vi "Clean_Up_Template.vi"(1 "Template Info In":string[](array[string])) -> (0 "Template Info Out":string[](array[string]))   [LabVIEW 2018]
uses:
  Controls/Global_mode.ctl
panel:
  in  "Mode":T1
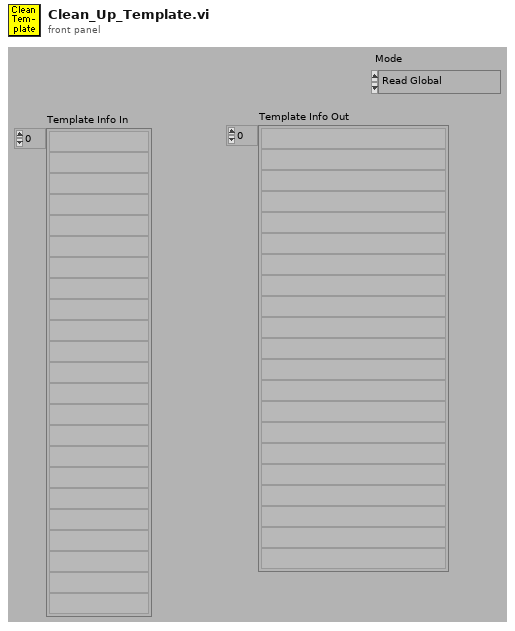
[diagram p1: front panel]
types:
  T1 = typedef "Global_mode.ctl" = enum16{"Read Global", "Load Global From File", "Write Global to File"}
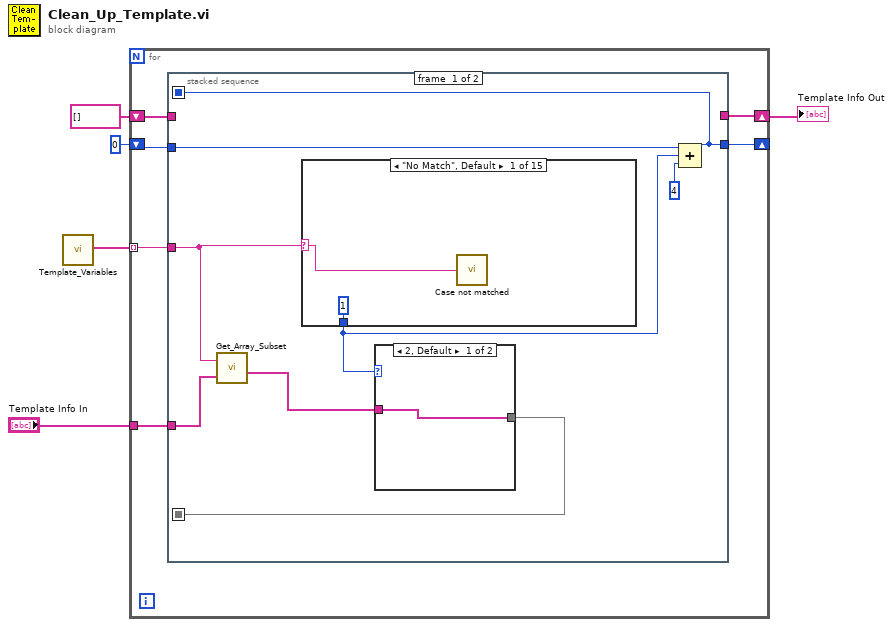
[diagram p0: block diagram]
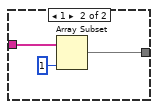
[diagram p2: hidden frame]
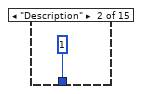
[diagram p3: hidden frame]
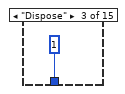
[diagram p4: hidden frame]
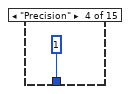
[diagram p5: hidden frame]
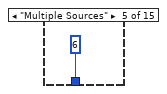
[diagram p6: hidden frame]
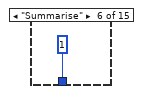
[diagram p7: hidden frame]
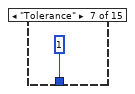
[diagram p8: hidden frame]
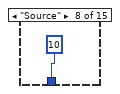
[diagram p9: hidden frame]
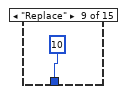
[diagram p10: hidden frame]
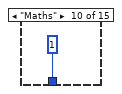
[diagram p11: hidden frame]
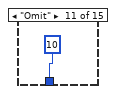
[diagram p12: hidden frame]
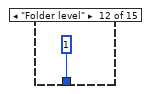
[diagram p13: hidden frame]
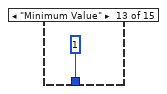
[diagram p14: hidden frame]
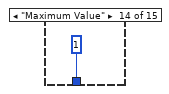
[diagram p15: hidden frame]
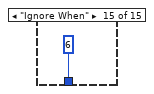
[diagram p16: hidden frame]
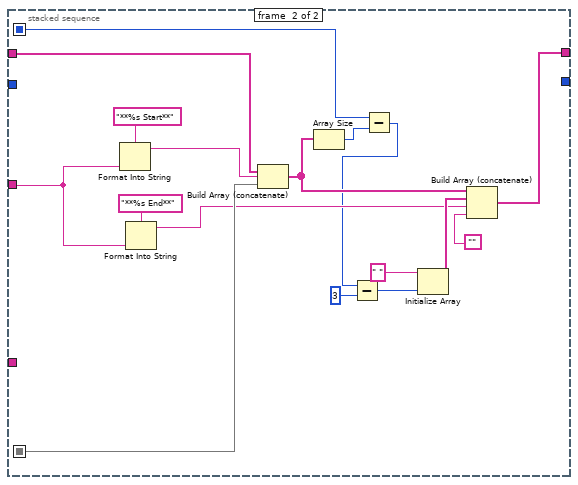
[diagram p17: hidden frame]
diagram:
  n1 = call "Template_Variables.vi"() -> ("Variable Names"=w1:string[])
  n2 = for {
    shift-right: [w6] -> w2
    shift-left: string[] [] -> [w7]
    tunnel: w1 -> [w11] mode=indexing
    tunnel: "Template Info In" -> [w10]
    shift-right: [w8] -> _
    shift-left: 0 -> [w9]
    n3 = stacked-sequence {
      seq-local: [w16 _] -> [_ w51]
      seq-local: [w12 _] -> [_ w49]
      tunnel: w11 -> [w18 w54]
      tunnel: w10 -> [w19 _]
      tunnel: w9 -> [w15 _]
      tunnel: [w12 _] -> w8
      tunnel: w7 -> [_ w53]
      tunnel: [_ w46] -> w6
      frame #0 {
        n4 = call "Get_Array_Subset.vi"("String Array In"=w19, "Subset Name"=w18) -> ("Array Subset Out"=w17:string[])  [unwired: 4 out]
        n5 = case shown="\"No Match\", Default" w18 {
          selector: w18 -> [w24 _ _ _ _ _ _ _ _ _ _ _ _ _ _]
          tunnel: [1 1 1 1 6 1 1 10 10 1 10 1 1 1 6] -> w14
          frame "No Match", Default {
            n6 = call "Case not matched.vi"("Case Name not Matched"=w24) -> ()
          }
          frame "Description" {
          }
          frame "Dispose" {
          }
          frame "Precision" {
          }
          frame "Multiple Sources" {
          }
          frame "Summarise" {
          }
          frame "Tolerance" {
          }
          frame "Source" {
          }
          frame "Replace" {
          }
          frame "Maths" {
          }
          frame "Omit" {
          }
          frame "Folder level" {
          }
          frame "Minimum Value" {
          }
          frame "Maximum Value" {
          }
          frame "Ignore When" {
          }
        }
        n7 = case shown="2, Default" w14 {
          tunnel: w17 -> [w20 w23]
          tunnel: [w20 w22] -> w16
          frame 2, Default {
          }
          frame 1 {
            n8 = Array Subset(array=w23, length=1 ("Array Length")) -> (w22:string[])  [unwired: 1 in]
          }
        }
        n9 = Compound Arithmetic op=ADD(w15, w14, 4) -> (w12:i32)
      }
      frame #1 {
        n10 = Format Into String(format string="**%s Start**" ("Format String"), w54) -> (resulting string=w52:string)  [unwired: 2 in, 1 out]
        n11 = Format Into String(format string="**%s End**" ("Format String"), w54) -> (resulting string=w44:string)  [unwired: 2 in, 1 out]
        n12 = Build Array (concatenate)(w53, w52, w51) -> (w48:string[])
        n13 = Array Size(array=w48) -> (size(s)=w50:i32)
        n14 = Subtract(x=w49, y=w50) -> (x-y=w43:i32)
        n15 = Subtract(x=w43, y=3) -> (x-y=w45:i32)
        n16 = Initialize Array(" ", w45) -> (w47:string[])
        n17 = Build Array (concatenate)(w48, w47, w44, "") -> (w46:string[])
      }
    }
  }
  "Template Info Out" <- w2
